vi "Close FP.vi"(8 "error in (no error)":errorcluster, 11 "VI in":refnum<vi>) -> (0 "error out":errorcluster)   [LabVIEW 2021, in "Pop-Up.lvlib" / "Popup.lvclass"]
doc: "Will close the front panel from the screen for the input VI Reference - should be used in all pop-up types that configure all the front panel BEFORE showing it when it is called so that the user doesn't see jitter\n\n<b>Code Developed By:</b> +\nDaniel Coons +\nhttps://github.com/danielcoons/tsc-pop-up"
uses:
  Popup.lvclass
  Popup.lvclass/Popup.ctl
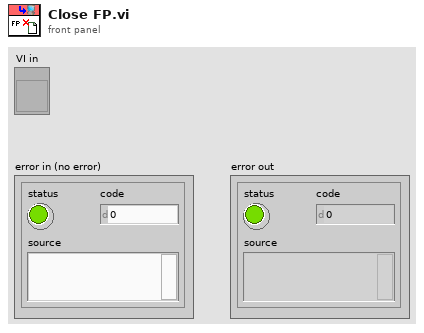
[diagram p1: front panel]
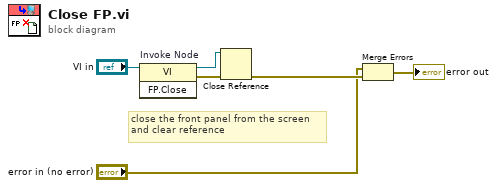
[diagram p0: block diagram]
diagram:
  # "close the front panel from the screen\nand clear reference"
  n1 = invoke on="Invoke Node" class="VI" method="FP.Close"(reference="VI in") -> (reference out=w5:refnum<vi>, error out=w4:errorcluster)  [unwired: 2 in, 1 out]
  n2 = Close Reference(reference=w5, error in (no error)=w4) -> (error out=w6:errorcluster)
  n3 = Merge Errors("error in (no error)", w6) -> (→"error out":errorcluster)
